vi "Error to Image.vi"(8 "error in (no error)":errorcluster, 11 "Image":T1) -> (3 "Image out":T1(plugin-control))   [LabVIEW 2016]
uses:
  <vilib>/vision/Image Controls.llb/IMAQ Image.ctl
  <vilib>/vision/NI_Vision_Development_Module.lvlib
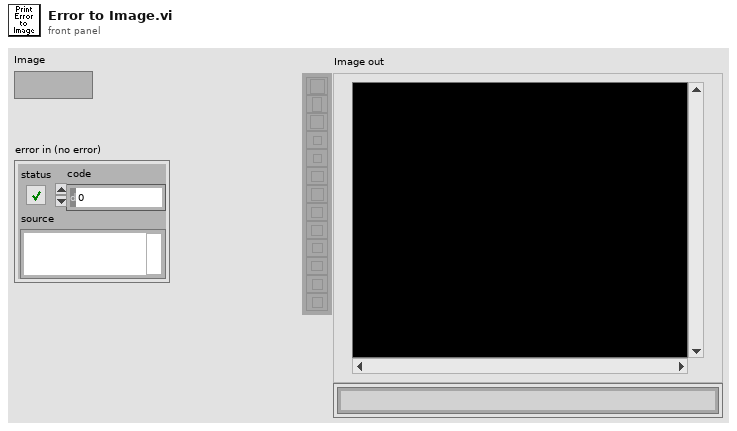
[diagram p1: front panel]
types:
  T1 = typedef "IMAQ Image.ctl" = refnum<image>
  T2 = cluster{"Desired Font (Application)":enum16{"User-specified Font", "Application Font", "System Font", "Dialog Font"}, "[User-specified Font]":cluster{"Font Name":string, "Size":i16, "Strikeout?":bool, "Italic?":bool, "Underline?":bool, "Outline?":bool, "Shadow?":bool, "Bold?":bool, "Rotation Angle":dbl}, "Horizontal Alignment":i16, "Vertical Alignment":i16}
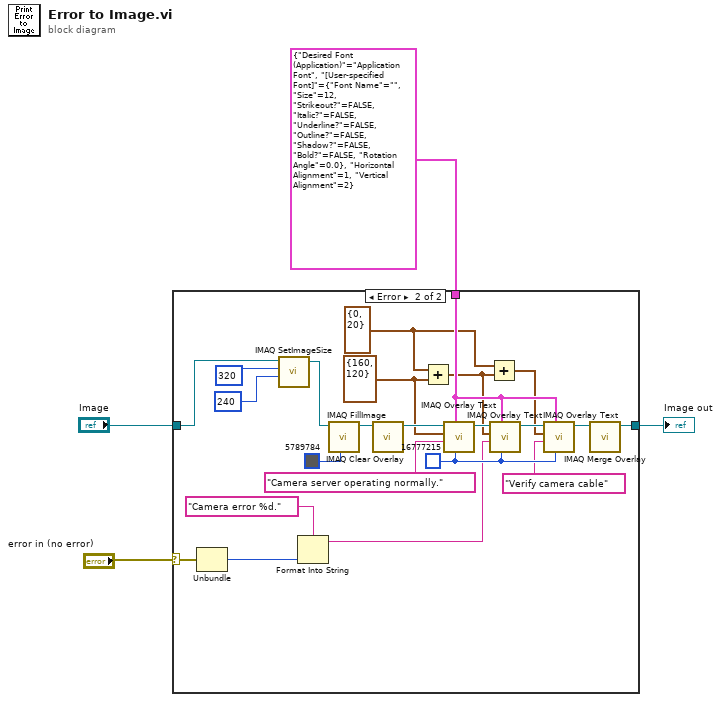
[diagram p0: block diagram]
diagram:
  n1 = case shown="Error" "error in (no error)" {
    selector: "error in (no error)" -> [_ w28]
    tunnel: "Image" -> [w5 w22]
    tunnel: [w5 w24] -> w2
    tunnel: T2 {"Desired Font (Application)"=enum."Application Font", "[User-specified Font]"={"Font Name"="", "Size"=12, "Strikeout?"=FALSE, "Italic?"=FALSE, "Underline?"=FALSE, "Outline?"=FALSE, "Shadow?"=FALSE, "Bold?"=FALSE, "Rotation Angle"=0.0}, "Horizontal Alignment"=1, "Vertical Alignment"=2} ("Font, Size & Style") -> [_ w15]
    frame No Error {
    }
    frame Error {
      w8 = cluster{"X":i32, "Y":i32} {"X"=0, "Y"=20} ("Origin")
      w14 = u32 16777215 ("Text Color (black)")
      w9 = cluster{"X":i32, "Y":i32} {"X"=160, "Y"=120} ("Origin")
      n2 = Unbundle(w28) -> ("code"=w23:i32)  [unwired: 2 out]
      n3 = call "IMAQ SetImageSize"("Y Resolution"=240, "X Resolution"=320, "Image"=w22) -> ("Image Out"=w19:T1)  [unwired: 2 in, 1 out]
      n4 = Format Into String(format string="Camera error %d.", w23) -> (resulting string=w11:string)  [unwired: 2 in, 1 out]
      n5 = call "IMAQ FillImage"("Color Pixel Value"=u32 5789784, "Image"=w19) -> ("Image Out"=w27:T1)  [unwired: 8 in, 1 out]
      n6 = call "IMAQ Clear Overlay"("Image"=w27) -> ("Image Out"=w26:T1)  [unwired: 9 in, 1 out]
      n7 = Add(x=w8, y=w9) -> (x+y=w6:cluster{"X":i32, "Y":i32})
      n8 = call "IMAQ Overlay Text"("Text Color (black)"=w14, "Font, Size & Style"=w15, "String"="Camera server operating normally.", "Origin"=w9, "Image"=w26) -> ("Image Out"=w18:T1)  [unwired: 5 in, 1 out]
      n9 = Add(x=w8, y=w6) -> (x+y=w7:cluster{"X":i32, "Y":i32})
      n10 = call "IMAQ Overlay Text"("Text Color (black)"=w14, "Font, Size & Style"=w15, "String"=w11, "Origin"=w6, "Image"=w18) -> ("Image Out"=w17:T1)  [unwired: 5 in, 1 out]
      n11 = call "IMAQ Overlay Text"("Text Color (black)"=w14, "Font, Size & Style"=w15, "String"="Verify camera cable", "Origin"=w7, "Image"=w17) -> ("Image Out"=w16:T1)  [unwired: 5 in, 1 out]
      n12 = call "IMAQ Merge Overlay"("Image Src"=w16) -> ("Image Dst Out"=w24:T1)  [unwired: 9 in, 1 out]
    }
  }
  "Image out" <- w2
